vi "VISA_ReadAndSave_4CHparalelos COM BUFFER DE LEITURA.vi"() -> ()   [LabVIEW 2019]
uses:
  813f916b-c519-439e-9418-14bd48b6d342.vi
  <vilib>/Instr/_visa.llb/VISA Configure Serial Port (Instr).vi
  <vilib>/Analysis/Matrix/Comparison/Not Equal/Not Equal.vi
  <vilib>/Analysis/Matrix/Comparison/Not Equal/Not Equal - RM,RM.vi
panel:
  in  "Tamanho do Buffer (leitura/plot)":i32=10
  out "loop time (ms)":dbl format="%.2f"
  out "Plot 3":dbl[](graph)
  out "Plot 2":dbl[](graph)
  out "Status Arquivo":errorcluster
  in  "file name":string
  out "Plot 1":dbl[](graph)
  out "Plot 0":dbl[](graph)
  out "Status Leitura":errorcluster
  out "Conversão Numérica":dbl[](array[numeric])
  out "Prévia da Leitura":string
  out "Status USB":errorcluster
  in  "Salvar Registro":bool
  in  "Gravando":bool
  in  "baud rate (115200)":u32=115200 caption="baud rate (9600)"
  in  "data bits (8)":u8=8 min=5 max=8 step=1
  in  "VISA resource name":refnum<visa-resource-name>="COM3"
  # "Controle de Salvamento"
  # "Log de Erros"
  # "Conversão Para Inteiro"
  # "Resultado da Leitura"
  # "Controle da porta Serial USB"
  # "Controle da Leitura"
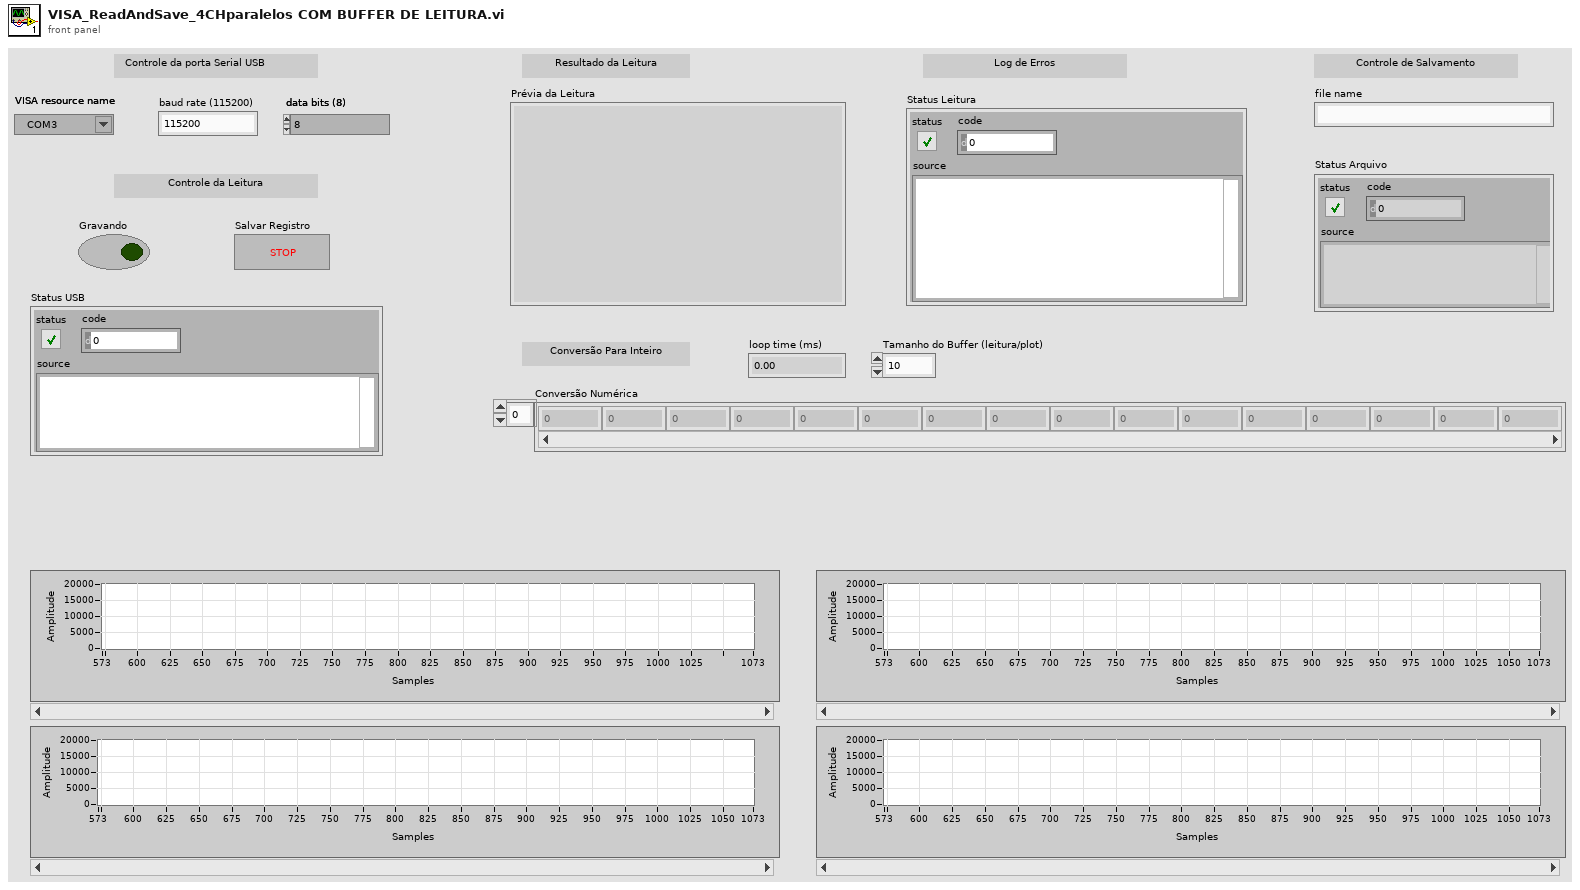
[diagram p1: front panel]
types:
  T1 = typedef "NI_Matrix.lvlib/RealMatrix.ctl" = dbl[][]
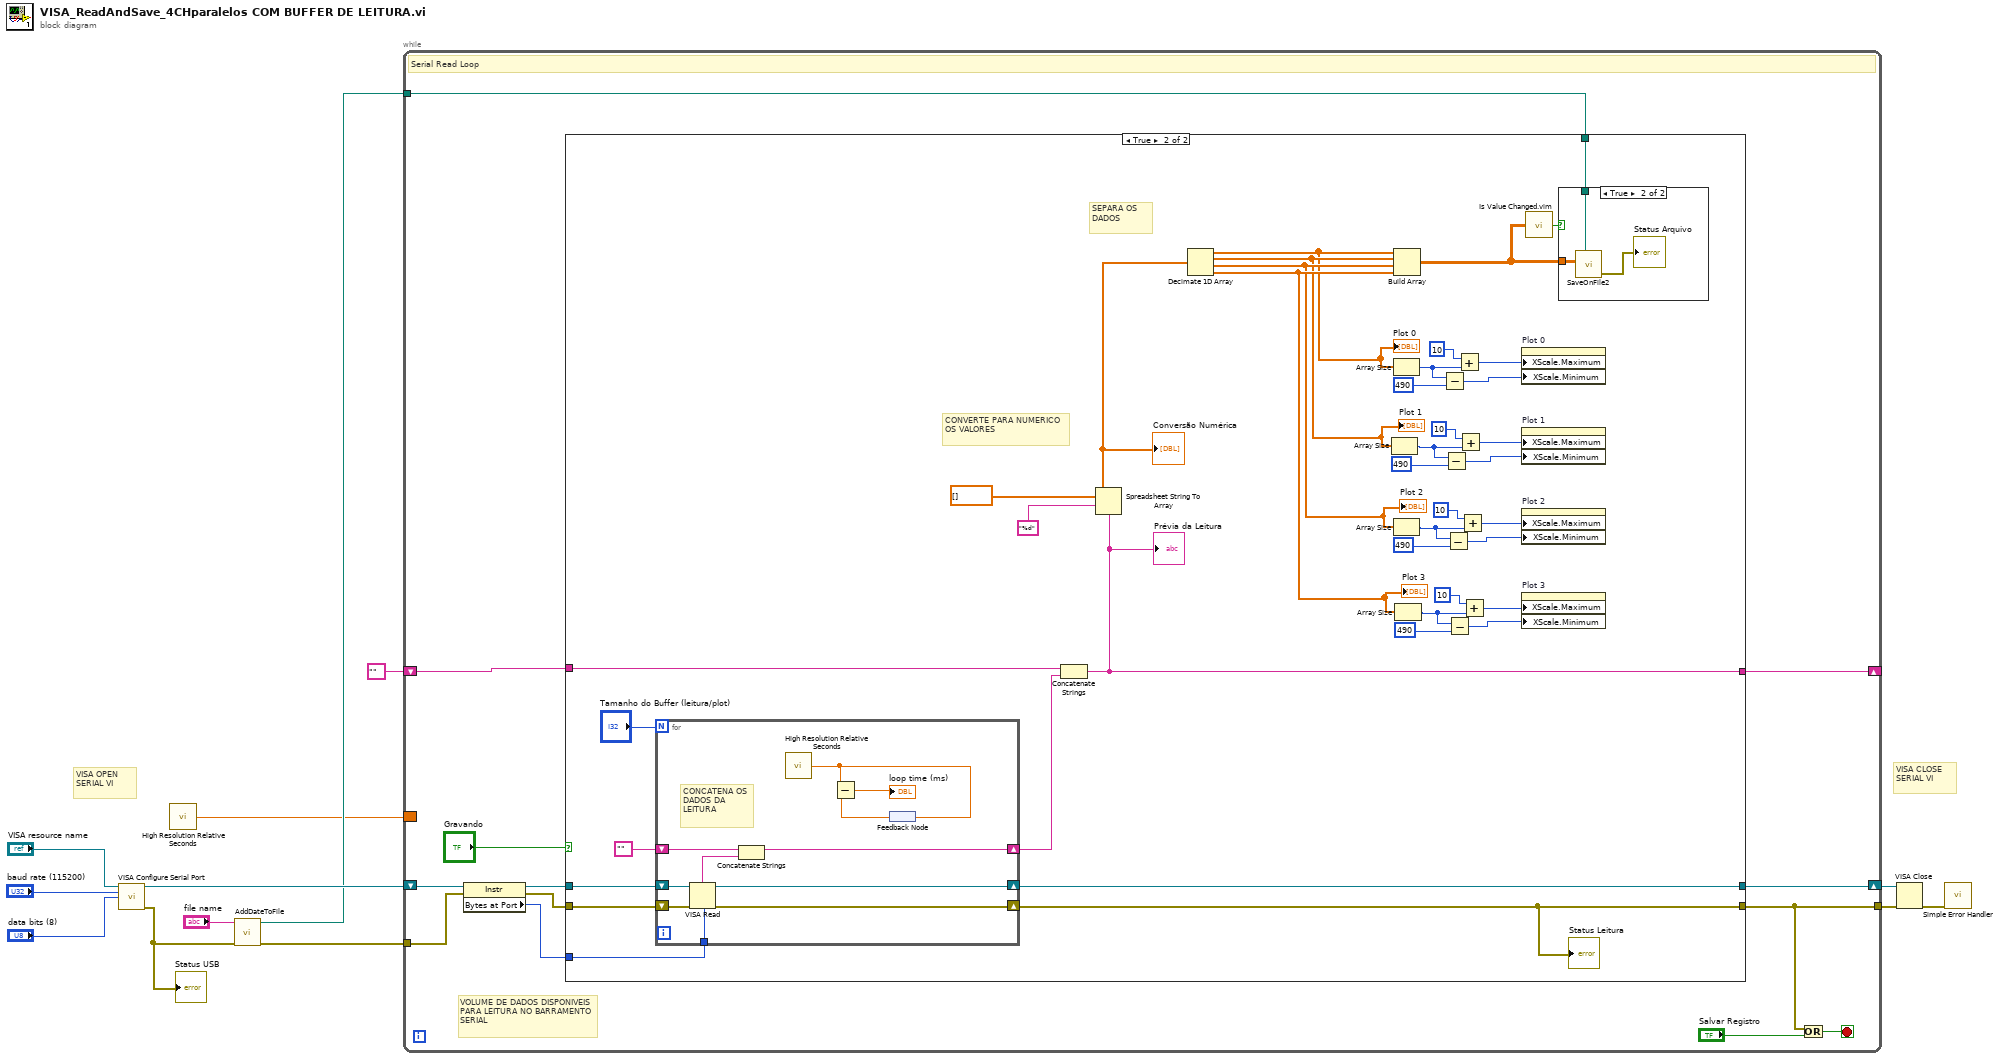
[diagram p0: block diagram]
diagram:
  # "VISA OPEN SERIAL VI"
  # "VISA CLOSE SERIAL VI"
  n1 = call-poly "VISA Configure Serial Port"("VISA resource name"="VISA resource name", "baud rate (9600)"="baud rate (115200)", "data bits (8)"="data bits (8)") -> ("VISA resource name out"=w11:refnum<visa-resource-name>, "error out"=w4:errorcluster)  [unwired: 11 in]
  "Status USB" <- w4
  n2 = call <vilib>:"High Resolution Relative Seconds.vi"() -> ("relative seconds"=w2:dbl)
  n3 = call "AddDateToFile.vi"("error in (no error)"=w4, "file name"="file name") -> ("error out"=w5:errorcluster, "new file path (Not A Path if cancelled)"=w3:path)  [unwired: 8 in]
  n4 = while {
    tunnel: w5 -> [w18]
    tunnel: [w24] -> w12
    shift-right: [w23] -> w10
    shift-left: w11 -> [w21]
    tunnel: w3 -> [w17]
    shift-right: [w15] -> _
    shift-left: "" -> [w16]
    border: w2 -> [_]
    stop <- w22 stop-if-true
    # "VOLUME DE DADOS DISPONIVEIS PARA LEITURA NO BARRAMENTO SERIAL"
    # "Serial Read Loop"
    n5 = property class="Instr"(reference=w21, error in=w18) -> (reference out=w19:refnum<visa-resource-name>, error out=w20:errorcluster, "Bytes at Port"=w14:u32)
    n6 = case shown="True" "Gravando" {
      tunnel: [w28 w35] -> w24
      tunnel: [w29 w34] -> w23
      tunnel: w19 -> [w29 w37]
      tunnel: w20 -> [w28 w36]
      tunnel: w17 -> [_ w61]
      tunnel: w16 -> [w27 w38]
      tunnel: [w27 w33] -> w15
      tunnel: w14 -> [_ w31]
      frame False {
        # "OS DADOS SÃO ACUMULADOS NO BUFFER ESPERANDO A PERMISSÃO PARA SER LIDOS"
      }
      frame True {
        # "SEPARA OS DADOS"
        # "CONVERTE PARA NUMERICO OS VALORES"
        n7 = for {
          N: "Tamanho do Buffer (leitura/plot)" -> [_]
          shift-right: [w79] -> w39
          shift-left: "" -> [w80]
          shift-right: [w75] -> w35
          shift-left: w36 -> [w76]
          shift-right: [w74] -> w34
          shift-left: w37 -> [w77]
          tunnel: w31 -> [w73]
          # "CONCATENA OS DADOS DA LEITURA"
          n8 = VISA Read(VISA resource name=w77, byte count=w73, error in (no error)=w76) -> (VISA resource name out=w74:refnum<visa-resource-name>, read buffer=w78:string, error out=w75:errorcluster)  [unwired: 1 out]
          n9 = Concatenate Strings(w80, w78) -> (w79:string)
          n10 = call <vilib>:"High Resolution Relative Seconds.vi"() -> ("relative seconds"=w71:dbl)
          n11 = feedback #1() -> (w70:dbl)
          n12 = Subtract(x=w71, y=w70) -> (x-y=→"loop time (ms)":dbl)
          n13 = feedback-in #1(w71) -> ()
        }
        "Status Leitura" <- w35
        n14 = Concatenate Strings(w38, w39) -> (w33:string)
        "Prévia da Leitura" <- w33
        n15 = Spreadsheet String To Array(format string="%d", spreadsheet string=w33, array type (2D Dbl)=dbl[] []) -> (array=w41:dbl[])  [unwired: 1 in]
        "Conversão Numérica" <- w41
        n16 = Decimate 1D Array(w41) -> (w42:dbl[], w43:dbl[], w44:dbl[], w45:dbl[])
        "Plot 0" <- w42
        "Plot 1" <- w43
        "Plot 2" <- w44
        "Plot 3" <- w45
        n17 = Array Size(array=w43) -> (size(s)=w57:i32)
        n18 = Array Size(array=w42) -> (size(s)=w64:i32)
        n19 = Array Size(array=w44) -> (size(s)=w54:i32)
        n20 = Build Array(w42, w43, w44, w45) -> (w32:T1)
        n21 = Array Size(array=w45) -> (size(s)=w51:i32)
        n22 = Subtract(x=w64, y=490) -> (x-y=w65:i32)
        n23 = Subtract(x=w57, y=490) -> (x-y=w60:i32)
        n24 = Subtract(x=w54, y=490) -> (x-y=w48:i32)
        n25 = Subtract(x=w51, y=490) -> (x-y=w46:i32)
        n26 = Add(x=10, y=w64) -> (x+y=w63:i32)
        n27 = Add(x=10, y=w57) -> (x+y=w59:i32)
        n28 = Add(x=10, y=w54) -> (x+y=w49:i32)
        n29 = Add(x=10, y=w51) -> (x+y=w47:i32)
        n30 = property on="Plot 0" class="WFGraph (strict)"("XScale.Maximum"=w63, "XScale.Minimum"=w65) -> ()  [unwired: 2 in, 2 out]
        n31 = property on="Plot 1" class="WFGraph (strict)"("XScale.Maximum"=w59, "XScale.Minimum"=w60) -> ()  [unwired: 2 in, 2 out]
        n32 = property on="Plot 2" class="WFGraph (strict)"("XScale.Maximum"=w49, "XScale.Minimum"=w48) -> ()  [unwired: 2 in, 2 out]
        n33 = property on="Plot 3" class="WFGraph (strict)"("XScale.Maximum"=w47, "XScale.Minimum"=w46) -> ()  [unwired: 2 in, 2 out]
        n34 = call "Is Value Changed.vim"("value"=w32) -> ("changed or first call?"=w67:bool)
        n35 = case shown="True" w67 {
          tunnel: w32 -> [_ w81]
          tunnel: w61 -> [_ w83]
          frame False {
          }
          frame True {
            n36 = call "SaveOnFile2.vi"("2D data"=w81, "file path (dialog if empty)"=w83) -> ("error file"=→"Status Arquivo":errorcluster)  [unwired: 5 in]
          }
        }
      }
    }
    n37 = Or(x=w24, y="Salvar Registro") -> (x .or. y?=w22:bool)
  }
  n38 = VISA Close(VISA resource name=w10, error in (no error)=w12) -> (error out=w9:errorcluster)
  n39 = call <vilib>:"Simple Error Handler.vi"("error in (no error)"=w9) -> ()  [unwired: 4 in, 5 out]
